vi "LVFunction_Imop_Compute_WavefrontParameters.vi"(0 "HasoData.lvclass":refnum<class "HasoData.lvclass">, 11 "error constant":errorcluster) -> (4 "HasoData.lvclass (dup)":refnum<class "HasoData.lvclass">, 6 "Parameters":T1, 15 "error out":errorcluster)   [LabVIEW 2020]
uses:
  HasoData.lvclass
  Geometric wavefront parameters.ctl
  LVClass_HasoData Read HasoData - property.vi
panel:
  out "tiltY":sgl
  out "tiltX":sgl
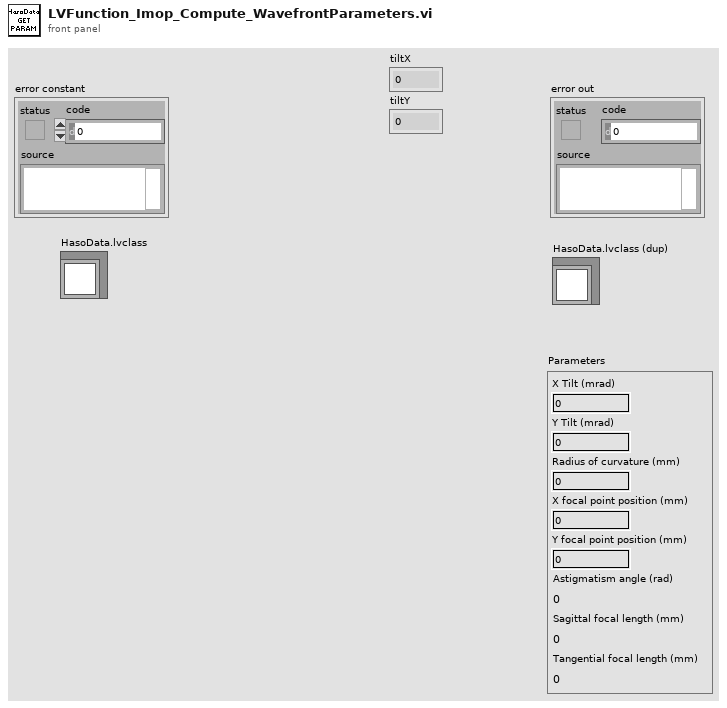
[diagram p1: front panel]
types:
  T1 = typedef "Geometric wavefront parameters.ctl" = cluster{"X Tilt (mrad)":sgl, "Y Tilt (mrad)":sgl, "Radius of curvature (mm)":sgl, "X focal point position (mm)":sgl, "Y focal point position (mm)":sgl, "Astigmatism angle (rad)":sgl, "Sagittal focal length (mm)":sgl, "Tangential focal length (mm)":sgl}
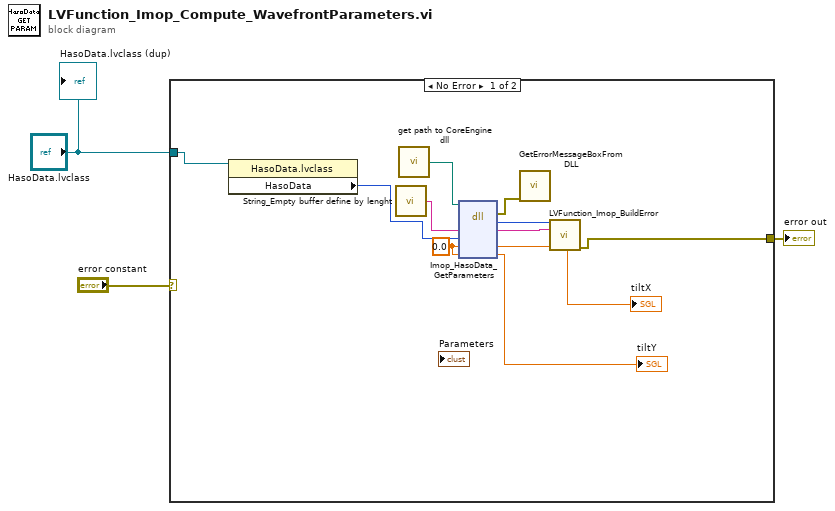
[diagram p0: block diagram]
diagram:
  n1 = case shown="No Error" "error constant" {
    selector: "error constant" -> [_ w15]
    tunnel: "HasoData.lvclass" -> [w9 _]
    tunnel: [w7 w15] -> w2
    frame No Error {
      w6 = sgl 0.0 ("tiltX")
      n2 = property class="HasoData.lvclass"(reference=w9) -> ("HasoData"=w8:i32)  [unwired: 1 in, 2 out]
      n3 = call "String_Empty buffer define by lenght.vi"() -> ("Empty buffer"=w12:string)  [unwired: 1 in]
      n4 = call "get path to CoreEngine dll.vi"() -> ("path to c_interface_vc100.dll"=w11:path)  [unwired: 12 in, 3 out]
      n5 = dll-call lib="D:/2_trunk/Soft_haso/ImOpCoreEngine4_LV2011/DLLs/ImopEngine4_vc100.dll" fn="Imop_HasoData_GetParameters"(path in=w11, "message"=w12, "HasoData"=w8, "tiltX"=w6, "tiltY"=w6) -> (error out=w10:errorcluster, "return type"=w14:i32, "message"=w13:string, "tiltX"=→"tiltX":sgl, "tiltY"=→"tiltY":sgl)  [unwired: 3 in, 1 out]
      n6 = call "GetErrorMessageBoxFromDLL.vi"("error IN"=w10) -> ()  [unwired: 10 in, 1 out]
      n7 = call "LVFunction_Imop_BuildError.vi"("code"=w14, "String to Prepend to source (\"\")"=w13) -> ("error out"=w7:errorcluster)  [unwired: 13 in]
    }
    frame Error {
    }
  }
  "error out" <- w2
  "HasoData.lvclass (dup)" <- "HasoData.lvclass"
